vi "fpga_LP2 Filter_coef0 (M Class_60Hz).vi"(0 "Memory In":refnum<k21>="coefROM", 2 "coefAddr":fxp<+,11,11>) -> (7 "coef":fxp<+/-,19,-3>, 9 "error":i32)   [LabVIEW 2013, in "NI_EP_PMU_FPGA.lvlib"]
uses:
  <vilib>/addons/Electrical Power/PMU/NI_EP_PMU_FPGA.lvlib
  <vilib>/rvi/Memory/Memory_Emulation/niFpgaMemoryEmulationReadFromVariant.vi
  <vilib>/rvi/Emulation/niFpgaSctlEmulationGetInTimedLoop.vi
  <vilib>/rvi/Memory/Memory_Emulation/niFpgaMemoryEmulationWriteToVariant.vi
  <vilib>/rvi/DataTransferAndStorage/Container/Common/niFpgaContainerExecOnDevCompGetState.vi
  <vilib>/rvi/DataTransferAndStorage/Container/Common/niFpgaContainerGetUniqueNameForEmu.vi
  <vilib>/rvi/errors/niFpgaSetErrorForExecOnDevCompSimple.vi
  <vilib>/rvi/Memory/Memory_Emulation/niFpgaMemoryEmulationCacheClearOnFirstRun.vi
  <vilib>/rvi/Memory/Memory_Emulation/nirvimemoryEmulationManagerCache_MakeExclusive.vi
  <vilib>/rvi/Memory/Memory_Emulation/niFpgaMemoryEmulationValidateCache.vi
  <vilib>/rvi/Memory/Memory_Emulation/nirvimemoryEmulationManagerCache_ReleaseExclusive.vi
  <vilib>/rvi/Memory/Memory_Emulation/nirvimemoryEmulationManagerCache_InsertValue.vi
  <vilib>/Utility/error.llb/Clear Errors.vi
  <vilib>/rvi/Memory/Memory_Emulation/nirvimemoryEmulationManagerCache_GetValue.vi
  <vilib>/rvi/DataTransferAndStorage/Container/XNode/niFpgaContainer.xnode
  <vilib>/rvi/Memory/Memory_Emulation/niFpgaMemoryEmulationRefIn.vi
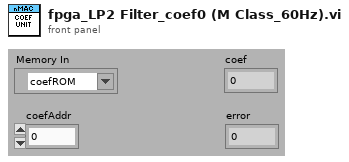
[diagram p1: front panel]
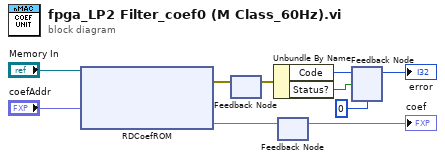
[diagram p0: block diagram]
diagram:
  n1 = xnode "RDCoefROM"("Address"="coefAddr", "Memory In"="Memory In") -> ("Data"=w8:fxp<+/-,19,-3>, "error out"=w6:errorcluster)  [unwired: 1 in, 1 out]
  n2 = feedback #1() -> (w5:errorcluster)  [unwired: 1 out]
  n3 = feedback-in #1(w6) -> ()
  n4 = Unbundle By Name(w5) -> ("Code"=w4:i32, "Status?"=w3:bool)
  n5 = feedback #2() -> (→"coef":fxp<+/-,19,-3>)  [unwired: 1 out]
  n6 = feedback-in #2(w8) -> ()
  n7 = feedback #3(0 ("Code")) -> (→"error":i32)
  n8 = feedback-in #3(w4, w3) -> ()
